vi "Get Valid Channels to Write.vi"(8 "error in (no error)":errorcluster, 9 "Data to Write In":cluster{waveform(dbl)[], string[]}, 10 "Stream Names In":string[](array[string]), 11 "Plugin in":refnum<class "StreamWriter.lvclass">) -> (0 "error out":errorcluster, 1 "Data to Write Out":cluster{waveform(dbl)[], string[]}, 2 "Stream Names Out":string[](array[string]), 3 "Plugin out":refnum<class "StreamWriter.lvclass">)   [LabVIEW 2024, in "StreamWriter.lvlib" / "StreamWriter.lvclass"]
uses:
  StreamWriter.lvclass
  <vilib>/FlexLogger/SDK/PluginSDK.lvlibp/PEFClasses/SDK/Plugin/Get Valid Consumer Channels.vi
  <vilib>/FlexLogger/SDK/PluginSDK.lvlibp/PEFClasses/SDK/Consumer Channel/Consumer Channel.lvclass
  StreamWriter.lvclass/StreamWriter.ctl
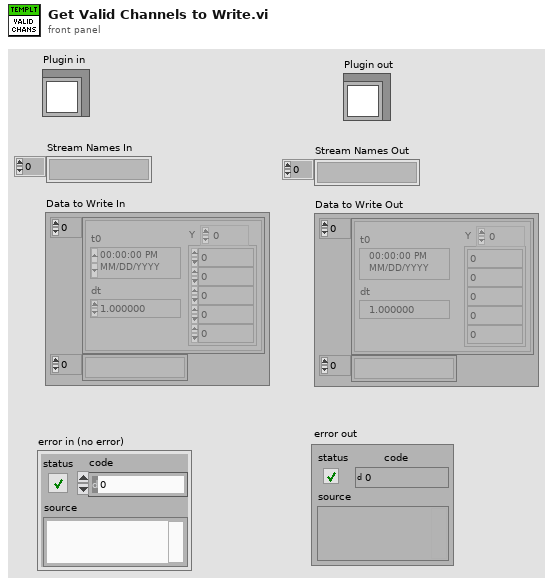
[diagram p1: front panel]
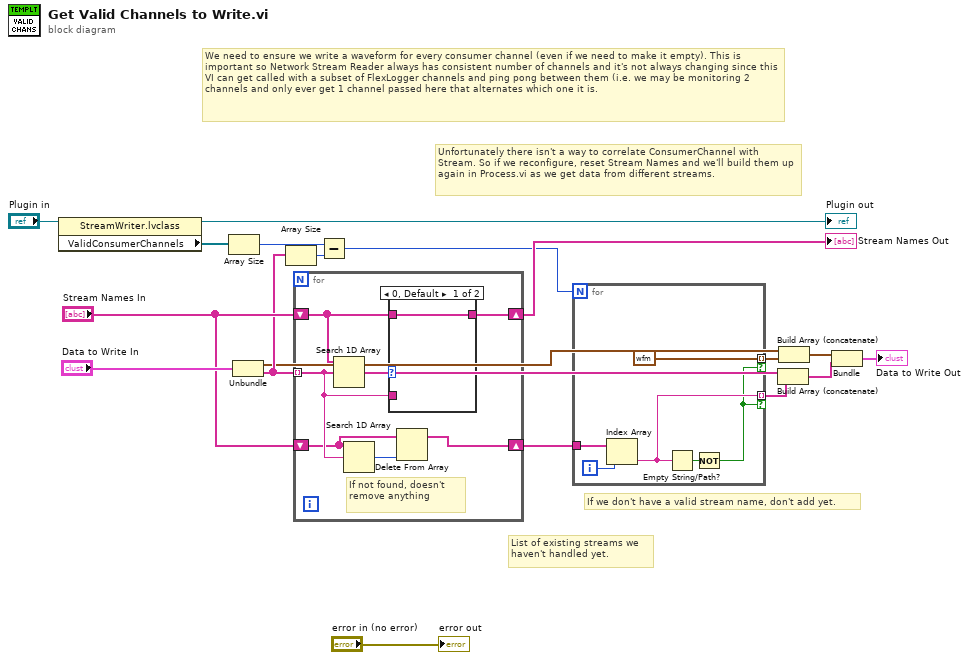
[diagram p0: block diagram]
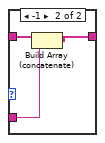
[diagram p2: hidden frame]
diagram:
  # "If we don't have a valid stream name, don't add yet."
  # "List of existing streams we haven't handled yet."
  # "Unfortunately there isn't a way to correlate ConsumerChannel with Stream. So if we reconfigure, reset Stream Names and we'll build them up again in Process.vi as we get data from different streams."
  # "We need to ensure we write a waveform for every consumer channel (even if we need to make it empty). This is important so Network Stream Reader always has consistent number of channels and it's not always changing since this VI can get called with a subset of FlexLogger channels and ping pong between them (i.e. we may be monitoring 2 channels and only ever get 1 channel passed here that alternates which one it is."
  n1 = property class="StreamWriter.lvclass"(reference="Plugin in") -> (reference out=→"Plugin out":refnum<class "StreamWriter.lvclass">, "ValidConsumerChannels"=w13:refnum<class "Consumer Channel.lvclass">[])  [unwired: 1 in, 1 out]
  n2 = Array Size(array=w13) -> (size(s)=w11:i32)
  n3 = Unbundle("Data to Write In") -> (w5:waveform(dbl)[], w7:string[])
  n4 = Array Size(array=w7) -> (size(s)=w10:i32)
  n5 = for {
    tunnel: w7 -> [w22] mode=indexing
    shift-right: [w23] -> w16
    shift-left: "Stream Names In" -> [w24]
    shift-right: [w19] -> w8
    shift-left: "Stream Names In" -> [w21]
    # "If not found, doesn't remove anything"
    n6 = Search 1D Array(1D array=w24, element=w22) -> (index of element=w25:i32)  [unwired: 1 in]
    n7 = Search 1D Array(1D array=w21, element=w22) -> (index of element=w20:i32)  [unwired: 1 in]
    n8 = case shown="0, Default" w25 {
      tunnel: w24 -> [w26 w29]
      tunnel: w22 -> [_ w28]
      tunnel: [w26 w27] -> w23
      frame 0, Default {
      }
      frame -1 {
        n9 = Build Array (concatenate)(w29, w28) -> (w27:string[])
      }
    }
    n10 = Delete From Array(array=w21, index=w20) -> (array with subset deleted=w19:string[])  [unwired: 1 in, 1 out]
  }
  "Stream Names Out" <- w16
  n11 = Subtract(x=w11, y=w10) -> (x-y=w9:i32)
  n12 = for {
    N: w9 -> [_]
    tunnel: w8 -> [w34]
    tunnel: [w32] -> w6 mode=indexing if=w30
    tunnel: [waveform(dbl) {"t0"=timestamp(0 s since 1904-01-01), "dt"=1.0, "Y"=[]} ("Waveform")] -> w4 mode=indexing if=w30
    i -> [w33]
    n13 = Index Array(array=w34, index=w33) -> (element=w32:string)
    n14 = Empty String/Path?(string/path=w32) -> (empty?=w31:bool)
    n15 = Not(x=w31) -> (.not. x?=w30:bool)
  }
  n16 = Build Array (concatenate)(w7, w6) -> (w2:string[])
  n17 = Build Array (concatenate)(w5, w4) -> (w3:waveform(dbl)[])
  n18 = Bundle(w3, w2) -> (→"Data to Write Out":cluster{waveform(dbl)[], string[]})  [unwired: 1 in]
  "error out" <- "error in (no error)"
